vi "Exit Module.vi"(8 "error in (no error)":errorcluster, 11 "Target Module":string) -> (0 "error out":errorcluster)   [LabVIEW 2020, in "CSM-FileSync.lvlib"]
uses:
  CSM-FileSync.lvlib
  <userlib>/_NEVSTOP/Communicable State Machine(CSM)/Communicable State Machine.lvlib
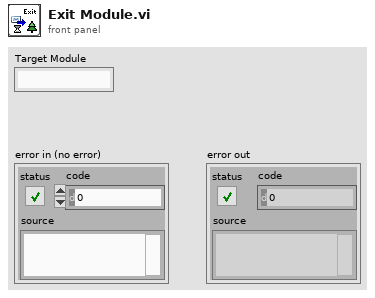
[diagram p1: front panel]
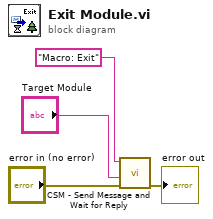
[diagram p0: block diagram]
diagram:
  n1 = call <userlib>:"CSM - Send Message and Wait for Reply.vi"("Error In (no error)"="error in (no error)", "Target Module"="Target Module", "State"="Macro: Exit") -> ("error out"=→"error out":errorcluster)  [unwired: 6 in, 2 out]
